vi "U-751 XY Stage Test Panel.vi"() -> ()   [LabVIEW 2016]
panel:
  in  "Quit":bool
  out "Stage Reply":string
  in  "Send Command":bool
  in  "Serial Command":string
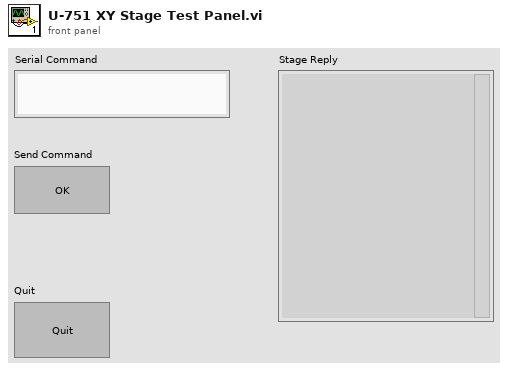
[diagram p1: front panel]
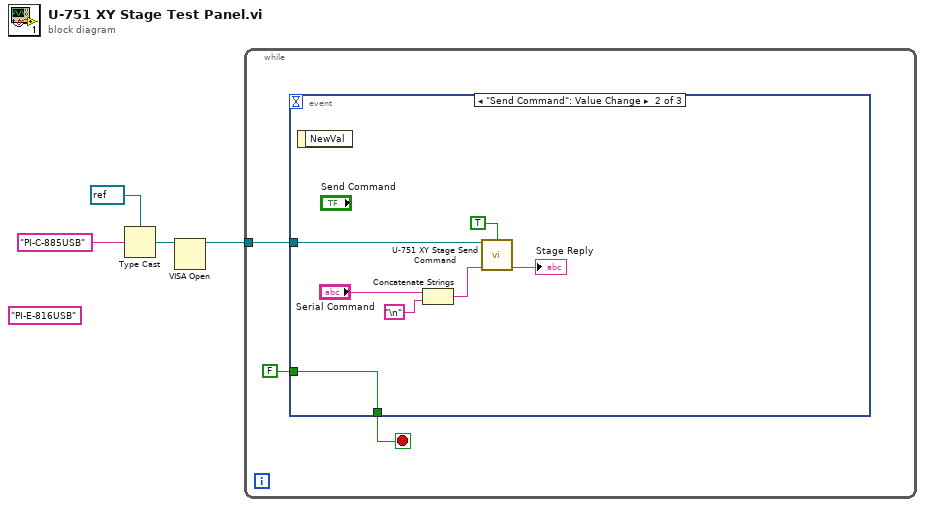
[diagram p0: block diagram]
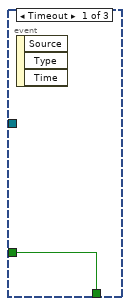
[diagram p2: hidden frame]
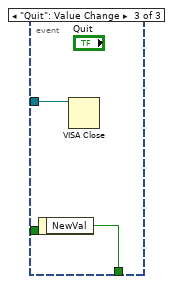
[diagram p3: hidden frame]
diagram:
  (unwired) "PI-E-816USB"
  n1 = Type Cast(type=refnum<visa-resource-name> refnum ("reference out"), x="PI-C-885USB") -> (*(type *) &x=w2:refnum<visa-resource-name>)
  n2 = VISA Open(VISA resource name=w2) -> (VISA resource name=w4:refnum<visa-resource-name>)  [unwired: 4 in, 1 out]
  n3 = while {
    tunnel: w4 -> [w5]
    stop <- w7 stop-if-true
    n4 = event shown="[1] \"Send Command\": Value Change" {
      selector: _ -> [_ _ _]
      dyn-events: _ -> [_ _ _]
      timeout: _ -> [_ _ _]
      tunnel: [w8 w15 w17] -> w7
      tunnel: FALSE -> [w8 w15 _]
      tunnel: w5 -> [_ w9 w16]
      event Timeout {
        n5 = event-data() -> ()  [unwired: 1 in, 3 out]
      }
      event "Send Command": Value Change {
        n6 = event-data() -> ()  [unwired: 1 in, 1 out]
        n7 = Concatenate Strings("Serial Command", "\n") -> (w12:string)
        n8 = call "U-751 XY Stage Send Command.vi"("VISA Ref"=w9, "Wait for Reply?"=TRUE, "Command"=w12) -> ("Response"=→"Stage Reply":string)  [unwired: 10 in, 2 out]
      }
      event "Quit": Value Change {
        n9 = event-data() -> ("NewVal"=w17:bool)  [unwired: 1 in]
        n10 = VISA Close(VISA resource name=w16) -> ()  [unwired: 1 in, 1 out]
      }
    }
  }
